vi "DeviceSendCommand.vi"(8 "error in (no error)":errorcluster, 9 "Data":variant, 10 "Command/Status":string, 11 "DeviceLoopData":T1) -> (0 "error out":errorcluster, 3 "DeviceLoopData Out":T1)   [LabVIEW 2014]
uses:
  DeviceLoopData.ctl
  NetworkStream/NetworkStreamData.ctl
  <vilib>/Utility/error.llb/Error Cluster From Error Code.vi
  <vilib>/ErrorRing/Error Ring.xnode
  NetworkStream/NetworkStream.lvlib
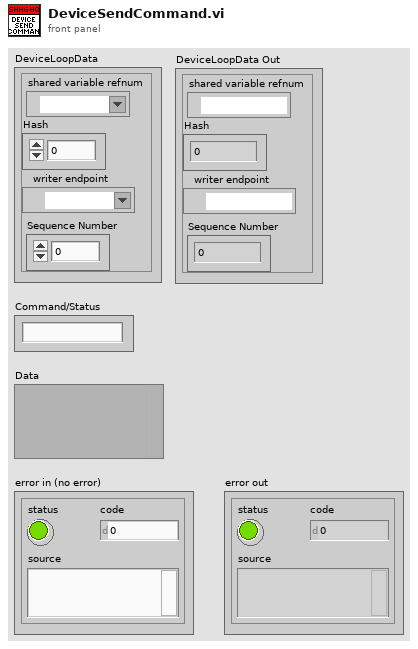
[diagram p1: front panel]
types:
  T1 = typedef "DeviceLoopData.ctl" = cluster{"shared variable refnum":refnum<k21>, "Hash":u64, "writer endpoint":refnum<k21>, "Sequence Number":u64}
  T2 = typedef "NetworkStream.lvlib/NetworkStreamData.ctl" = cluster{"Command/Status":string, "Data":variant, "Session Hash":u64, "Sequence Number":u64}
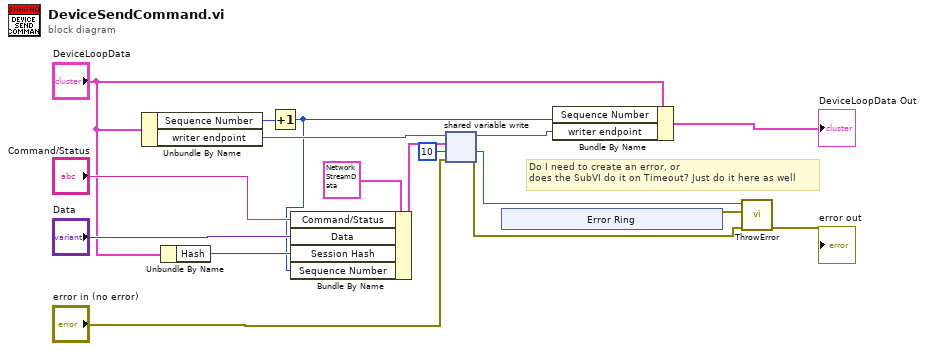
[diagram p0: block diagram]
diagram:
  # "Do I need to create an error, or \ndoes the SubVI do it on Timeout? Just do it here as well"
  n1 = Unbundle By Name("DeviceLoopData") -> ("Sequence Number"=w2:u64, "writer endpoint"=w3:refnum<k21>)
  n2 = Unbundle By Name("DeviceLoopData") -> ("Hash"=w6:u64)
  n3 = Increment(x=w2) -> (x+1=w1:u64)
  n4 = Bundle By Name(cluster=T2 {"Command/Status"="Random Number", "Data"=variant, "Session Hash"=0, "Sequence Number"=0} ("data in"), "Command/Status"="Command/Status", "Data"="Data", "Session Hash"=w6, "Sequence Number"=w1) -> (w4:T2)
  n5 = shared-variable-write(w3, "error in (no error)", w4, 10 ("timeout ms (-1)")) -> (w5:refnum<k21>, w9:errorcluster, w11:bool)
  n6 = xnode "Error Ring"() -> ("error out"=w10:errorcluster)
  n7 = Bundle By Name(cluster="DeviceLoopData", "Sequence Number"=w1, "writer endpoint"=w5) -> (→"DeviceLoopData Out":T1)
  n8 = call "ThrowError.vi"("error in (no error)"=w9, "current error in"=w10, "Boolean"=w11) -> ("error out"=→"error out":errorcluster)  [unwired: 8 in]
